vi "WriteGraph(SubVI).vi"(8 "Error In":errorcluster, 9 "ComboBox in":refnum<vi>, 10 "Arr Refnum":refnum<vi>, 11 "XYGraph in":refnum<vi>) -> (0 "Error Out":errorcluster)   [LabVIEW 2018]
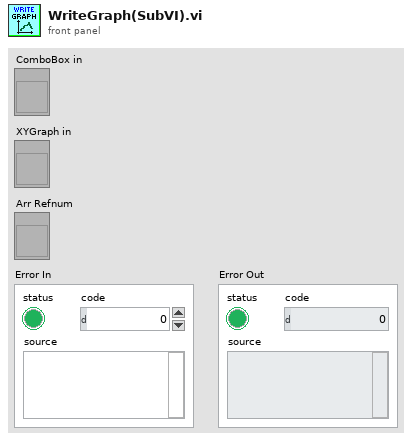
[diagram p1: front panel]
types:
  T1 = typedef "LVComboBoxStrsAndValuesArrayTypeDef.ctl" = cluster{"String":string, "Value":string}[]
  T2 = typedef "Line.ctl" = cluster{"Width":dbl, "Color":i64, "Array Oy":dbl[], "Array Ox":dbl[], "Name":string, "Plot Visible":T3}
  T3 = typedef "View.ctl" = bool
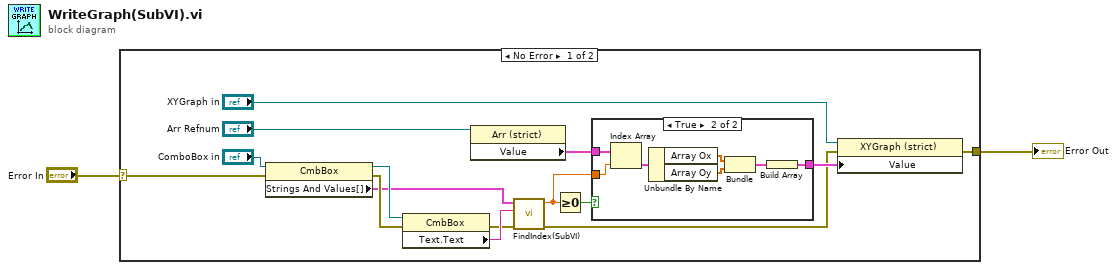
[diagram p0: block diagram]
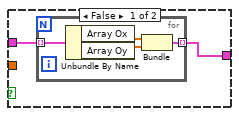
[diagram p2: hidden frame]
diagram:
  n1 = case shown="No Error" "Error In" {
    selector: "Error In" -> [w15 w31]
    tunnel: [w3 w31] -> w1
    frame No Error {
      n2 = property on="Property Node" class="CmbBox"(reference="ComboBox in", error in=w15) -> (reference out=w13:refnum<vi>, error out=w12:errorcluster, "Strings And Values[]"=w11:T1)
      n3 = property on="Property Node" class="CmbBox"(reference=w13, error in=w12) -> (error out=w7:errorcluster, "Text.Text"=w10:string)  [unwired: 1 out]
      n4 = property on="Property Node" class="Arr (strict)"(reference="Arr Refnum") -> ("Value"=w8:T2[])  [unwired: 1 in, 2 out]
      n5 = call "FindIndex(SubVI).vi"("Error In"=w7, "Name"=w10, "Strings And Values[]"=w11) -> ("Error Out"=w4:errorcluster, "Index"=w6:dbl)  [unwired: 7 in]
      n6 = Greater Or Equal To 0?(x=w6) -> (x >= 0?=w9:bool)
      n7 = case shown="True" w9 {
        tunnel: w8 -> [w19 w30]
        tunnel: w6 -> [_ w29]
        tunnel: [w18 w24] -> w5
        frame False {
          n8 = for {
            tunnel: w19 -> [w23] mode=indexing
            tunnel: [w20] -> w18 mode=indexing
            n9 = Unbundle By Name(w23) -> ("Array Ox"=w22:dbl[], "Array Oy"=w21:dbl[])
            n10 = Bundle("Array Ox"=w22, "Array Oy"=w21) -> (w20:cluster{"Array Ox":dbl[], "Array Oy":dbl[]})  [unwired: 1 in]
          }
        }
        frame True {
          n11 = Index Array(array=w30, index=w29) -> (element=w28:T2)
          n12 = Unbundle By Name(w28) -> ("Array Ox"=w27:dbl[], "Array Oy"=w26:dbl[])
          n13 = Bundle("Array Ox"=w27, "Array Oy"=w26) -> (w25:cluster{"Array Ox":dbl[], "Array Oy":dbl[]})  [unwired: 1 in]
          n14 = Build Array(w25) -> (w24:cluster{"Array Ox":dbl[], "Array Oy":dbl[]}[])
        }
      }
      n15 = property on="Property Node" class="XYGraph (strict)"(reference="XYGraph in", error in=w4, "Value"=w5) -> (error out=w3:errorcluster)  [unwired: 1 out]
    }
    frame Error {
    }
  }
  "Error Out" <- w1
